vi "runSaveScripts.vi"(8 "error in (no error)":errorcluster, 11 "ScriptListCompiler in":refnum<class "ScriptListCompiler.lvclass">) -> (0 "error out":errorcluster, 3 "ScriptListCompiler out":refnum<class "ScriptListCompiler.lvclass">)   [LabVIEW 2009, in "Compiler.lvlib" / "ScriptListCompiler.lvclass"]
uses:
  ScriptListCompiler.lvclass
  Filing/FileSystem/FileSystem.lvclass
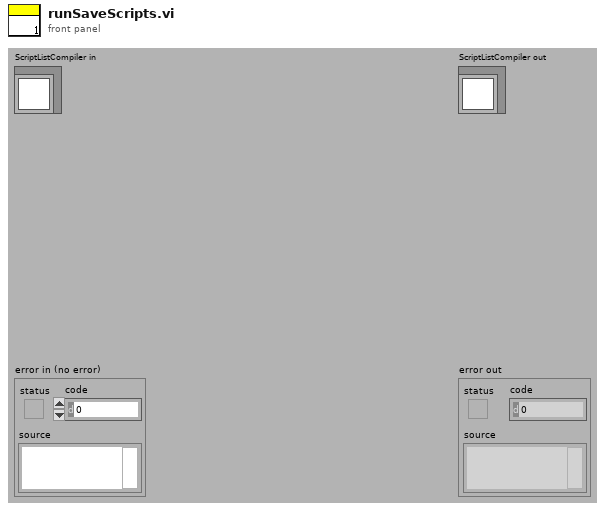
[diagram p1: front panel]
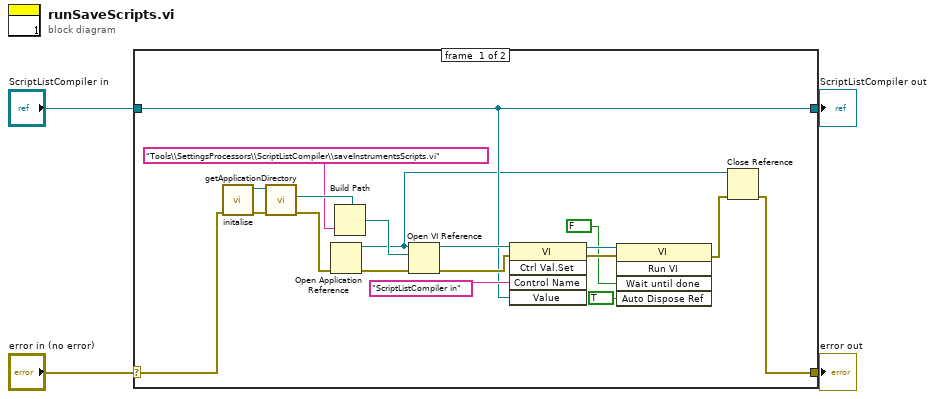
[diagram p0: block diagram]
diagram:
  n1 = case shown="No Error" "error in (no error)" {
    selector: "error in (no error)" -> [w17 w25]
    tunnel: [w5 w25] -> w3
    tunnel: [w12 w24] -> w1
    tunnel: "ScriptListCompiler in" -> [w12 w24]
    frame #0 {
      n2 = call "initalise.vi"("error in (no error)"=w17) -> ("error out"=w21:errorcluster, "FileSystem out"=w22:refnum<class "FileSystem.lvclass">)  [unwired: 9 in]
      n3 = call-dynamic "getApplicationDirectory.vi"("error in (no error)"=w21, "FileSystem.lvclass in"=w22) -> ("error out"=w18:errorcluster, "ApplicationDirectory"=w19:path)  [unwired: 7 in, 1 out]
      n4 = Open Application Reference(8:w18) -> (0:w23:errorcluster, 3:w7:refnum<vi>)  [unwired: 3 in]
      n5 = Build Path(base path=w19, name or relative path="Tools\\SettingsProcessors\\ScriptListCompiler\\saveInstrumentsScripts.vi") -> (appended path=w20:path)
      n6 = Open VI Reference(application reference (local)=w7, vi path=w20, error in (no error)=w23) -> (vi reference=w15:refnum<vi>, error out=w14:errorcluster)  [unwired: 3 in]
      n7 = invoke class="VI" method="Ctrl Val.Set"(reference=w15, error in=w14, "Control Name"="ScriptListCompiler in", "Value"=w12) -> (reference out=w10:refnum<vi>, error out=w11:errorcluster)  [unwired: 1 in, 3 out]
      n8 = invoke class="VI" method="Run VI"(reference=w10, error in=w11, "Wait until done"=FALSE, "Auto Dispose Ref"=TRUE ("Auto Dispose Reference")) -> (error out=w6:errorcluster)  [unwired: 1 in, 4 out]
      n9 = Close Reference(reference=w7, error in (no error)=w6) -> (error out=w5:errorcluster)
    }
    frame #1 {
    }
  }
  "error out" <- w3
  "ScriptListCompiler out" <- w1
